vi "FrequencyConversion.vi"(10 "Command Echo":u8[](array[numeric]), 11 "Scalar":dbl) -> (1 "Waveform Graph":u16[](graph), 2 "detected frequency":dbl format="%.2p", 3 "Tuner Recommendation":string)   [LabVIEW 2019]
uses:
  <vilib>/measure/matone.llb/Extract Single Tone Information 1 Chan.vi
  <vilib>/measure/NI_MAPro.lvlib
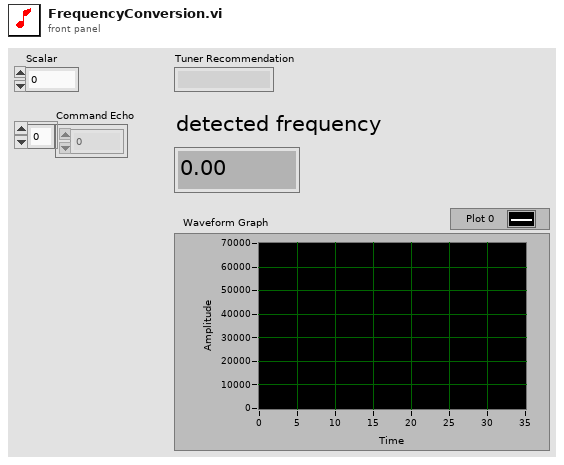
[diagram p1: front panel]
types:
  T1 = enum16{"big-endian, network order", "native, host order", "little-endian"}
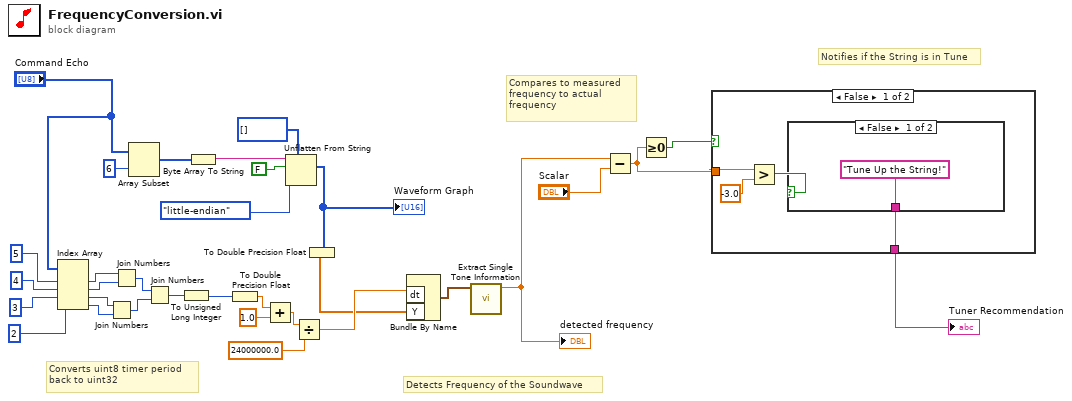
[diagram p0: block diagram]
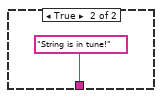
[diagram p2: hidden frame]
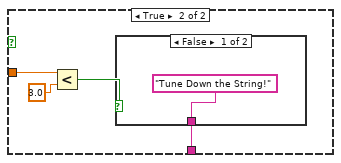
[diagram p3: hidden frame]
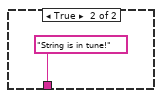
[diagram p4: hidden frame]
diagram:
  # "Compares to measured \nfrequency to actual\nfrequency"
  # "Notifies if the String is in Tune"
  # "Detects Frequency of the Soundwave"
  # "Converts uint8 timer period \nback to uint32"
  n1 = Index Array(array="Command Echo", index #1=5 ("index"), index #2=4 ("index"), index #3=3 ("index"), index #4=2 ("index")) -> (element #1=w12:u8, element #2=w13:u8, element #3=w14:u8, element #4=w15:u8)
  n2 = Join Numbers(hi=w14, lo=w15) -> ((hi.lo)=w16:u16)
  n3 = Join Numbers(hi=w12, lo=w13) -> ((hi.lo)=w17:u16)
  n4 = Array Subset(array="Command Echo", index=6) -> (w2:u8[])  [unwired: 1 in]
  n5 = Join Numbers(hi=w17, lo=w16) -> ((hi.lo)=w18:u32)
  n6 = To Unsigned Long Integer(number=w18) -> (unsigned 32bit integer=w22:u32)
  n7 = Byte Array To String(unsigned byte array=w2) -> (string=w3:string)
  n8 = To Double Precision Float(number=w22) -> (double precision float=w23:dbl)
  n9 = Add(x=w23, y=1.0) -> (x+y=w25:dbl)
  n10 = Unflatten From String(type=u16[] [], binary string=w3, data includes array or string size? (T)=FALSE, byte order (0:big-endian, network order)=T1."little-endian") -> (value=w11:u16[])  [unwired: 1 in, 2 out]
  "Waveform Graph" <- w11
  n11 = Divide(x=w25, y=24000000.0) -> (x/y=w27:dbl)
  n12 = To Double Precision Float(number=w11) -> (double precision float=w8:dbl[])
  n13 = Bundle By Name("dt"=w27, "Y"=w8) -> (w7:waveform(dbl))  [unwired: 1 in]
  n14 = call-poly <vilib>:"Extract Single Tone Information.vi"("time signal in"=w7) -> ("detected frequency"=w32:dbl)  [unwired: 5 in, 5 out]
  "detected frequency" <- w32
  n15 = Subtract(x=w32, y="Scalar") -> (x-y=w30:dbl)
  n16 = Greater Or Equal To 0?(x=w30) -> (x >= 0?=w29:bool)
  n17 = case shown="False" w29 {
    tunnel: w30 -> [w34 w41]
    tunnel: [w36 w39] -> w31
    frame False {
      n18 = Greater?(x=w34, y=-3.0) -> (0:w33:bool)
      n19 = case shown="False" w33 {
        tunnel: ["Tune Up the String!" ("Tuner Recommendation") "String is in tune!" ("Tuner Recommendation")] -> w36
        frame False {
        }
        frame True {
        }
      }
    }
    frame True {
      n20 = Less?(x=w41, y=3.0) -> (x < y?=w42:bool)
      n21 = case shown="False" w42 {
        tunnel: ["Tune Down the String!" ("Tuner Recommendation") "String is in tune!" ("Tuner Recommendation")] -> w39
        frame False {
        }
        frame True {
        }
      }
    }
  }
  "Tuner Recommendation" <- w31
